vi "MainGUI.vi"(8 "ErrorIn":errorcluster, 11 "TAFTraceWindowIn":refnum<class "TAFTraceWindow.lvclass">) -> ()   [LabVIEW 2021, in "TAFTraceWindow.lvclass"]
uses:
  TAFTraceWindow.lvclass
  C:/Localdata/Projects/TriekselSoft/TriekselsoftApplicationFramework/Source/.Externals/Library_YAF/YActor/YActor.lvclass
  TAFTraceWindow_UiCallBackEvents.ctl
  TAFTraceWindow.lvclass/TAFTraceWindow.ctl
  <vilib>/Utility/miscctls.llb/LVRowAndColumnUnsignedTypeDef.ctl
  TAFTraceWindow_ClassCast.vi
  Library_YAF/YActor/YActor.lvclass
  C:/Localdata/Projects/TriekselSoft/TriekselsoftApplicationFramework/Source/.Externals/Library_YAF/YAFTAF/YAFTAF.lvclass
  C:/Localdata/Projects/TriekselSoft/TriekselsoftApplicationFramework/Source/.Externals/Interface_UserInterface_IFrontPanel/IFrontPanel/IFrontPanel.lvclass
  C:/Localdata/Projects/TriekselSoft/TriekselsoftApplicationFramework/Source/IInterface/IInterface.lvclass
  C:/Localdata/Projects/TriekselSoft/TriekselsoftApplicationFramework/Source/.Externals/Interface_Object_ICreateDestroy/ICreateDestroy/ICreateDestroy.lvclass
  C:/Localdata/Projects/TriekselSoft/TriekselsoftApplicationFramework/Source/.Externals/Interface_Object_IPersistentData/IPersistentData/IPersistentData.lvclass
  C:/Localdata/Projects/TriekselSoft/TriekselsoftApplicationFramework/Source/.Externals/Interface_TAF_ITAFObject/ITAFObject/ITAFObject.lvclass
  C:/Localdata/Projects/TriekselSoft/TriekselsoftApplicationFramework/Source/.Externals/Library_TAF_TraceWindow/TAFTraceWindow/TAFTraceWindow.lvclass
  C:/Localdata/Projects/TriekselSoft/TriekselsoftApplicationFramework/Source/.Externals/INewOpenCVMat/INewOpenCVMat.lvclass
  C:/Localdata/Projects/TriekselSoft/TriekselsoftApplicationFramework/Source/.Externals/Interface_TAF_TraceSubscriptor/ITAFFilteredTrace/ITAFFilteredTrace.lvclass
panel:
  in  "Size":i32=1000 format="%d lines"
  out "L_busy":i32
  out "Trace":string[][](table)
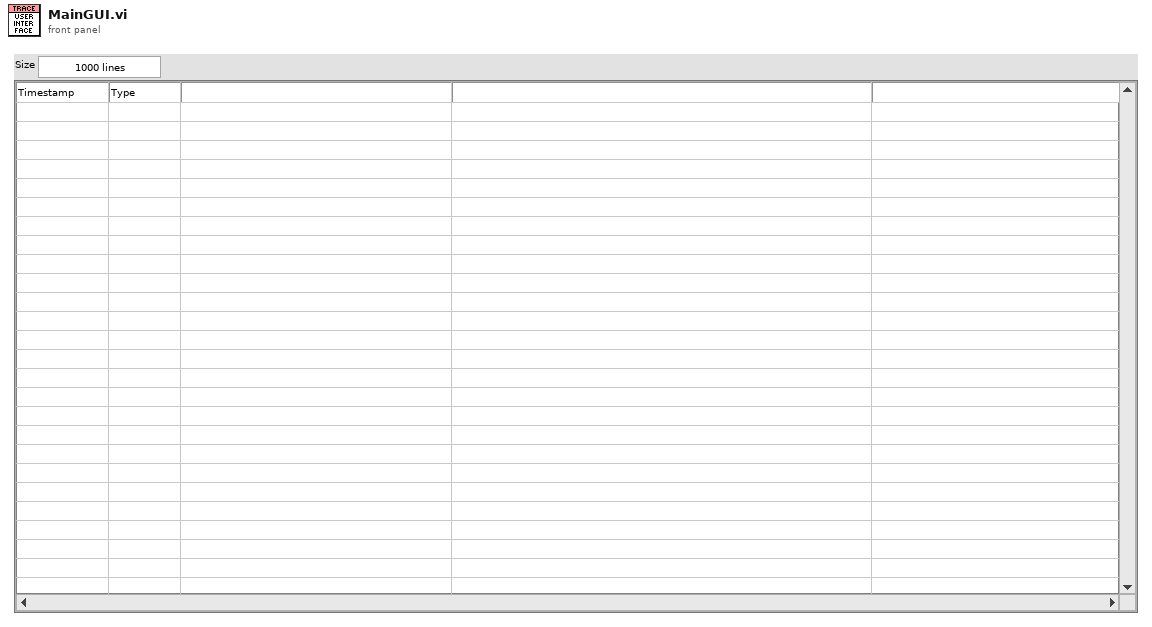
[diagram p1: front panel]
types:
  T1 = enum32{"Invalid", "Standard", "Closed", "Hidden", "Minimized", "Maximized"}
  T2 = typedef "TAFTraceWindow.lvclass/TAFTraceWindow_UiCallBackEvents.ctl" = enum16{"Default", "PersistentDataUpdated"}
  T3 = cluster{"Event":string, "This":refnum<class>, "Data":variant}
  T4 = typedef "LVRowAndColumnUnsignedTypeDef.ctl" = cluster{"Row":u32, "Column":u32}
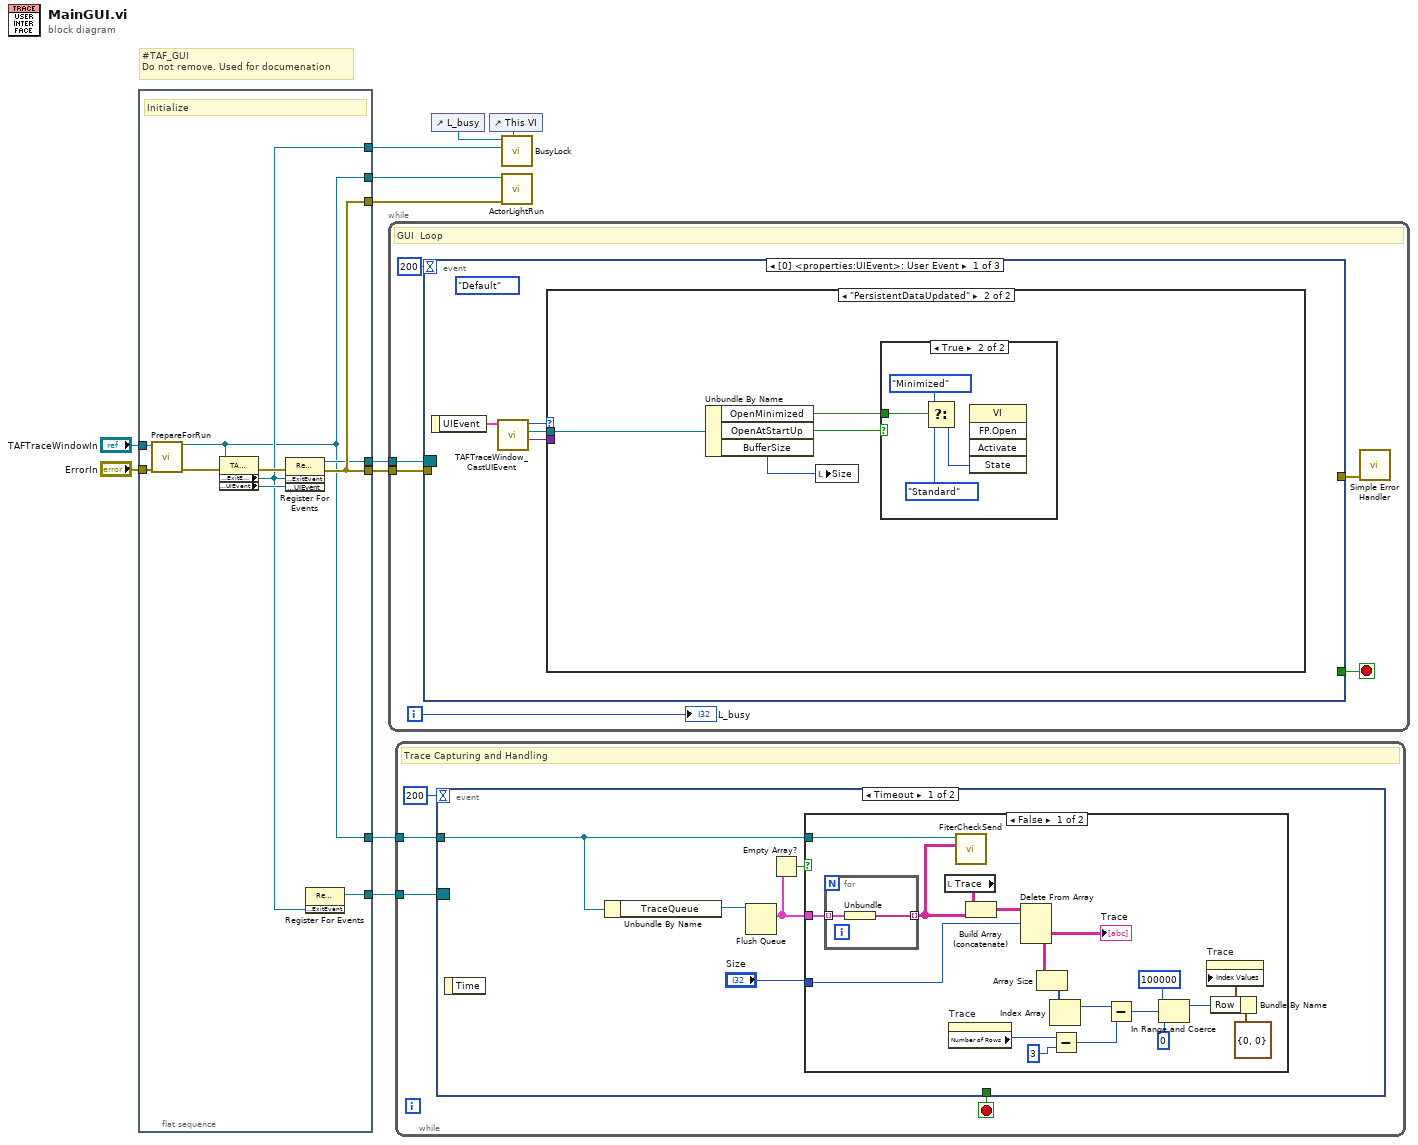
[diagram p0: block diagram]
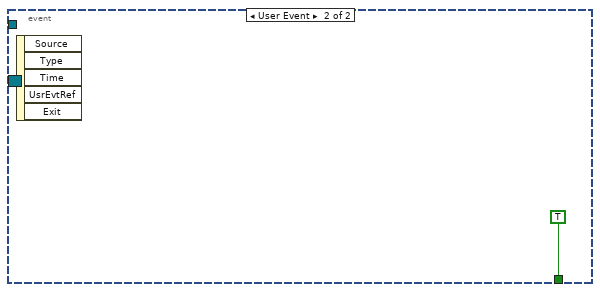
[diagram p3: hidden frame]
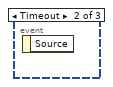
[diagram p6: hidden frame]
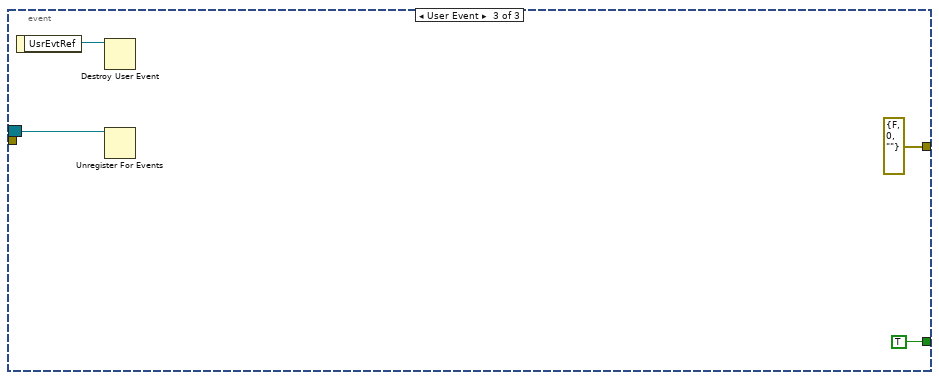
[diagram p7: hidden frame]
diagram:
  # "#TAF_GUI\nDo not remove. Used for documenation"
  n1 = flat-sequence {
    tunnel: "ErrorIn" -> [w21]
    tunnel: "TAFTraceWindowIn" -> [w17]
    tunnel: [w16] -> w7
    tunnel: [w13] -> w4
    tunnel: [w18] -> w10
    tunnel: [w12] -> w3
    tunnel: [w18] -> w9
    tunnel: [w14] -> w2
    tunnel: [w12] -> w1
    frame #0 {
      # "Initialize"
      n2 = call-dynamic "PrepareForRun.vi"("ErrorIn"=w21, "YActorIn"=w17) -> ("ErrorOut"=w19:errorcluster, "YActorOut"=w12:refnum<class "TAFTraceWindow.lvclass">)  [unwired: 8 in]
      n3 = property class="TAFTraceWindow"(reference=w12, error in=w19) -> (error out=w20:errorcluster, "properties:ExitEvent"=w13:refnum<user-event>, "properties:UIEvent"=w15:refnum<user-event>)  [unwired: 1 out]
      n4 = register-events(error in=w20, w13, w15) -> (reference out=w16:refnum<event-registration>, error out=w18:errorcluster)  [unwired: 1 in]
      n5 = register-events(w13) -> (reference out=w14:refnum<event-registration>)  [unwired: 2 in, 1 out]
    }
  }
  n6 = while {
    tunnel: w10 -> [w27]
    tunnel: w7 -> [w24]
    i -> [w23]
    stop <- w25 stop-if-true
    # "GUI  Loop"
    n7 = event shown="[0] <properties:UIEvent>: User Event" {
      selector: w24 -> [_ _ w41]
      dyn-events: _ -> [_ _ _]
      timeout: 200 -> [_ _ _]
      tunnel: w27 -> [_ _ _]
      tunnel: [_ _ TRUE] -> w25
      tunnel: [_ _ errorcluster {"Status"=FALSE, "Code"=0, "Source"=""} ("ErrorOut")] -> w26
      event User Event {
        (unwired) TAFTraceWindow_UiCallBackEvents."Default" ("UiEventNames")
        n8 = event-data() -> ("UIEvent"=w31:T3)  [unwired: 1 in]
        n9 = call "TAFTraceWindow_CastUIEvent.vi"("UIEvent"=w31) -> ("Data"=w28:variant, "ApplicationGUIOut"=w29:refnum<class "TAFTraceWindow.lvclass">, "UiEventNames"=w30:T2)  [unwired: 8 in]
        n10 = case shown="\"PersistentDataUpdated\"" w30 {
          tunnel: w29 -> [_ w33]
          tunnel: w28 -> [_ _]
          frame Default {
          }
          frame "PersistentDataUpdated" {
            n11 = Unbundle By Name(w33) -> ("OpenMinimized"=w34:bool, "OpenAtStartUp"=w35:bool, "BufferSize"=w32:i32)
            n12 = local write "Size"(w32) -> ()
            n13 = case shown="True" w35 {
              tunnel: w34 -> [_ w39]
              frame False {
              }
              frame True {
                n14 = Select(t=T1."Minimized" ("State"), s=w39, f=T1."Standard" ("State")) -> (s? t:f=w36:T1)
                n15 = invoke class="VI" method="FP.Open"("State"=w36) -> ()  [unwired: 4 in, 5 out]
              }
            }
          }
        }
      }
      event Timeout {
        n16 = event-data() -> ()  [unwired: 1 in, 1 out]
      }
      event User Event {
        n17 = event-data() -> ("UsrEvtRef"=w40:refnum<user-event>)  [unwired: 1 in]
        n18 = Destroy User Event(user event=w40) -> ()  [unwired: 1 in, 1 out]
        n19 = Unregister For Events(event registration refnum=w41) -> ()  [unwired: 1 in, 1 out]
      }
    }
    n20 = call <vilib>:"Simple Error Handler.vi"("error in (no error)"=w26) -> ()  [unwired: 4 in, 5 out]
    "L_busy" <- w23
  }
  n21 = while {
    tunnel: w2 -> [w47]
    tunnel: w1 -> [w45]
    stop <- w46 stop-if-true
    # "Trace Capturing and Handling"
    n22 = event shown="[0] Timeout" {
      selector: w47 -> [_ _]
      dyn-events: _ -> [_ _]
      timeout: 200 -> [_ _]
      tunnel: [_ TRUE] -> w46
      tunnel: w45 -> [w48 _]
      event Timeout {
        n23 = event-data() -> ()  [unwired: 1 in, 1 out]
        n24 = Unbundle By Name(w48) -> ("TraceQueue"=w52:refnum<queue>)
        n25 = Flush Queue(queue=w52) -> (remaining elements=w50:cluster{string[]}[])  [unwired: 1 in, 2 out]
        n26 = Empty Array?(array=w50) -> (empty?=w49:bool)
        n27 = case shown="False" w49 {
          tunnel: "Size" -> [w68 _]
          tunnel: w50 -> [w67 _]
          tunnel: w48 -> [w53 _]
          frame False {
            n28 = for {
              tunnel: w67 -> [w72] mode=indexing
              tunnel: [w71] -> w54 mode=indexing
              n29 = Unbundle(w72) -> (w71:string[])
            }
            n30 = local read "Trace"() -> (w70:string[][])
            n31 = property on="Trace" class="Tbl (strict)"() -> ("Number of Rows"=w57:u32)  [unwired: 2 in, 2 out]
            n32 = call "FiterCheckSend.vi"("TraceData"=w54, "TAFTraceWindow in"=w53) -> ()  [unwired: 10 in]
            n33 = Build Array (concatenate)(w70, w54) -> (w69:string[][])
            n34 = Delete From Array(array=w69, length=w68) -> (deleted portion=w58:string[][])  [unwired: 2 in, 1 out]
            "Trace" <- w58
            n35 = Array Size(array=w58) -> (size(s)=w64:i32[])
            n36 = Index Array(array=w64) -> (element=w63:i32)  [unwired: 1 in]
            n37 = Subtract(x=w57, y=u32 3) -> (x-y=w55:u32)
            n38 = Subtract(x=w63, y=w55) -> (x-y=w59:u32)
            n39 = In Range and Coerce(upper limit=100000, x=w59, lower limit=0) -> (coerced(x)=w62:u32)  [unwired: 1 out]
            n40 = Bundle By Name(cluster=T4 {"Row"=0, "Column"=0} ("Index Values"), "Row"=w62) -> (w65:T4)
            n41 = property on="Trace" class="Tbl (strict)"("Index Values"=w65) -> ()  [unwired: 2 in, 2 out]
          }
          frame True {
          }
        }
      }
      event User Event {
        n42 = event-data() -> ()  [unwired: 1 in, 5 out]
      }
    }
  }
  n43 = control-ref of="L_busy"() -> (w6:refnum<vi>)
  n44 = control-ref of="This VI"() -> (w5:refnum<vi>)
  n45 = call "BusyLock.vi"("BusyLock"=w5, "ExitEvent"=w4, "Counter"=w6) -> ()  [unwired: 9 in]
  n46 = call "ActorLightRun.vi"("ErrorIn"=w9, "YActorIn"=w3) -> ()  [unwired: 8 in, 2 out]
